vi "_Set Item Property.vi"(6 "Set as BinaryString (F)":bool, 8 "error in (no error)":errorcluster, 9 "Value":variant, 10 "Property Name":string, 11 "Item Ref in":T1 format="%.0x") -> (0 "error out":errorcluster, 3 "Item Ref out":T1 format="%.0x", 4 "Replaced":bool)   [LabVIEW 2020, in "Custom Device API.lvlib"]
uses:
  <vilib>/NI VeriStand/Custom Device API/Custom Device API.lvlib
  <vilib>/NI VeriStand/Custom Device API/Custom Device Item Ref.ctl
  ea0f6146-6498-45d2-a045-41a514eb0288.vi
  <vilib>/NI VeriStand/Custom Device API/Custom Device Offline Path.vi
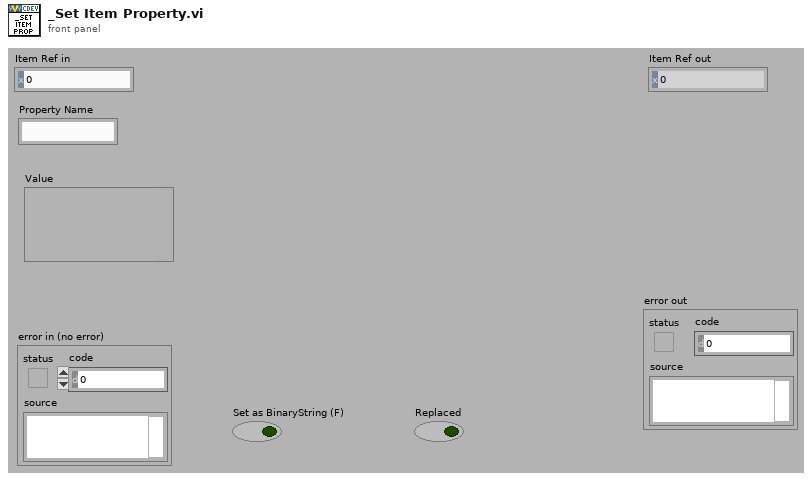
[diagram p1: front panel]
types:
  T1 = typedef "Custom Device API.lvlib/Custom Device Item Ref.ctl" = u64
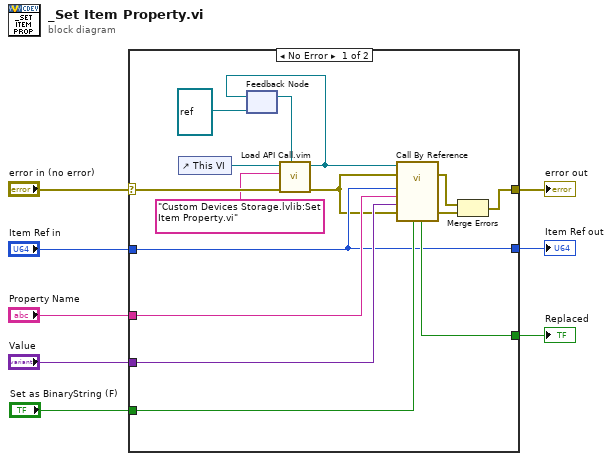
[diagram p0: block diagram]
diagram:
  n1 = case shown="No Error" "error in (no error)" {
    selector: "error in (no error)" -> [w13 w24]
    tunnel: "Set as BinaryString (F)" -> [w23 _]
    tunnel: [w22 _] -> w7
    tunnel: [w16 w25] -> w6
    tunnel: [w21 w24] -> w5
    tunnel: "Value" -> [w20 _]
    tunnel: "Property Name" -> [w19 _]
    tunnel: "Item Ref in" -> [w16 w25]
    frame No Error {
      n2 = control-ref of="This VI"() -> (w14:refnum<vi>)
      n3 = feedback #1(refnum<vi> refnum ("type specifier VI Refnum (for type only)")) -> (w15:refnum<vi>)
      n4 = call "Load API Call.vim"("VI reference in"=w15, "error in (no error)"=w13, "VI qualified name"="Custom Devices Storage.lvlib:Set Item Property.vi", "Caller VI ref"=w14) -> ("error out"=w11:errorcluster, "VI reference"=w12:refnum<vi>)  [unwired: 6 in]
      n5 = feedback-in #1(w12) -> ()
      n6 = call-by-ref "?"(reference=w12, error in=w11, "Set as BinaryString"=w23, 8:"error in (no error)"=w11, "Value"=w20, "Property Name"=w19, "Item Ref in"=w16) -> (error out=w18:errorcluster, 0:"error out"=w17:errorcluster, "Replaced"=w22:bool)  [unwired: 4 in, 2 out]
      n7 = Merge Errors(w18, w17) -> (w21:errorcluster)
    }
    frame Error {
    }
  }
  "Replaced" <- w7
  "Item Ref out" <- w6
  "error out" <- w5
